vi "Event Demo Sub Close.vi"(2 "stop":refnum<vi>, 3 "error in":errorcluster, 4 "exit counter":refnum<vi>, 5 "sub vi references":T1) -> (0 "error out":errorcluster)   [LabVIEW 2019]
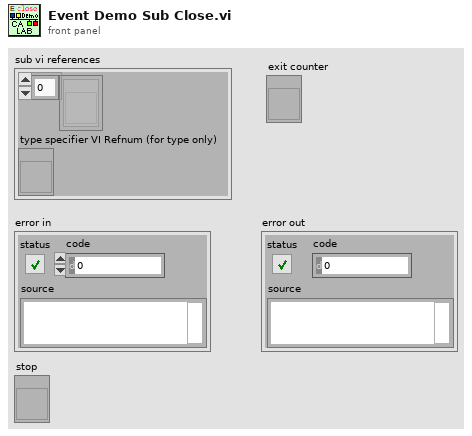
[diagram p1: front panel]
types:
  T1 = cluster{refnum<vi>[], "type specifier VI Refnum (for type only)":refnum<vi>}
  T2 = enum8{"Enabled", "Disabled", "Disabled and Grayed Out"}
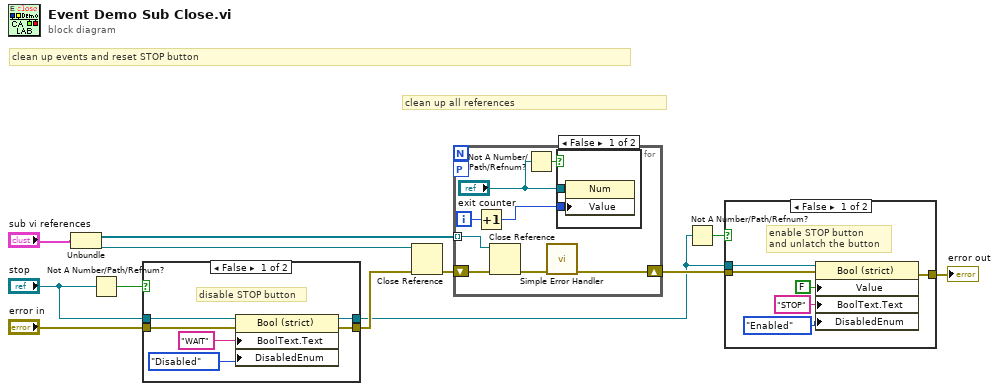
[diagram p0: block diagram]
diagram:
  # "clean up all references"
  # "clean up events and reset STOP button"
  n1 = Unbundle("sub vi references") -> (w8:refnum<vi>[], "type specifier VI Refnum (for type only)"=w7:refnum<vi>)
  n2 = Not A Number/Path/Refnum?(number/path/refnum="stop") -> (NaN/Path/Refnum?=w5:bool)
  n3 = case shown="False" w5 {
    tunnel: [w16 w20] -> w9
    tunnel: "error in" -> [w15 w20]
    tunnel: "stop" -> [w14 w19]
    tunnel: [w13 w19] -> w2
    frame False {
      # "disable STOP button"
      n4 = property class="Bool (strict)"(reference=w14, error in=w15, "BoolText.Text"="WAIT" ("Boolean Text.Text"), "DisabledEnum"=T2."Disabled" ("Disabled")) -> (reference out=w13:refnum<vi>, error out=w16:errorcluster)
    }
    frame True {
    }
  }
  n5 = Close Reference(reference=w7, error in (no error)=w9) -> (error out=w11:errorcluster)
  n6 = for {
    shift-right: [w21] -> w12
    shift-left: w11 -> [w28]
    tunnel: w8 -> [w26] mode=indexing
    workers-P: _ -> [_]
    i -> [w25]
    n7 = Increment(x=w25) -> (x+1=w24:i32)
    n8 = Close Reference(reference=w26, error in (no error)=w28) -> (error out=w27:errorcluster)
    n9 = Not A Number/Path/Refnum?(number/path/refnum="exit counter") -> (NaN/Path/Refnum?=w23:bool)
    n10 = call <vilib>:"Simple Error Handler.vi"("error in (no error)"=w27) -> ("error out"=w21:errorcluster)  [unwired: 4 in, 4 out]
    n11 = case shown="False" w23 {
      tunnel: "exit counter" -> [w30 _]
      tunnel: w24 -> [w29 _]
      frame False {
        n12 = property class="Num"(reference=w30, "Value"=w29) -> ()  [unwired: 1 in, 2 out]
      }
      frame True {
      }
    }
  }
  n13 = Not A Number/Path/Refnum?(number/path/refnum=w2) -> (NaN/Path/Refnum?=w4:bool)
  n14 = case shown="False" w4 {
    tunnel: w12 -> [w36 w37]
    tunnel: [w35 w37] -> w10
    tunnel: w2 -> [w31 _]
    frame False {
      # "enable STOP button\nand unlatch the button"
      n15 = property class="Bool (strict)"(reference=w31, error in=w36, "Value"=FALSE, "BoolText.Text"="STOP" ("Label.Text"), "DisabledEnum"=T2."Enabled" ("Disabled")) -> (error out=w35:errorcluster)  [unwired: 1 out]
    }
    frame True {
    }
  }
  "error out" <- w10
